vi "data_load_display_trend_fft_mea_coll_v5.vi"() -> ()   [LabVIEW 2020]
uses:
  <vilib>/Utility/file.llb/Read Delimited Spreadsheet (DBL).vi
panel:
  in  "Numeric 2":i32
  out "Waveform Graph 2":dbl[][](graph)
  out "Spectrum plot 2":cluster{i32, dbl, "spectrum out":dbl[]}(graph)
  out "Frequency Interval: delta(f) 2":dbl
  out "xf (frequency) 2":dbl[](array[numeric])
  out "size(s) 2":i32
  out "df (Hz) 2":dbl
  out "ploted signal from each selected frequency 2":dbl[][](graph)
  out "signal from each selected frequency 2":dbl[][](array[numeric])
  out "phase 3":dbl[](array[numeric])
  out "magnitude 3":dbl[](array[numeric])
  out "Numeric 4":i32
  out "Time vs Acceleration graph 2":cluster{"all rows":dbl[], "all rows":dbl[]}(graph)
  out "Acceleration 2":dbl[](array[numeric])
  out "time 2":dbl[](array[numeric])
  out "array w/ subset deleted 2":dbl[][](array[numeric])
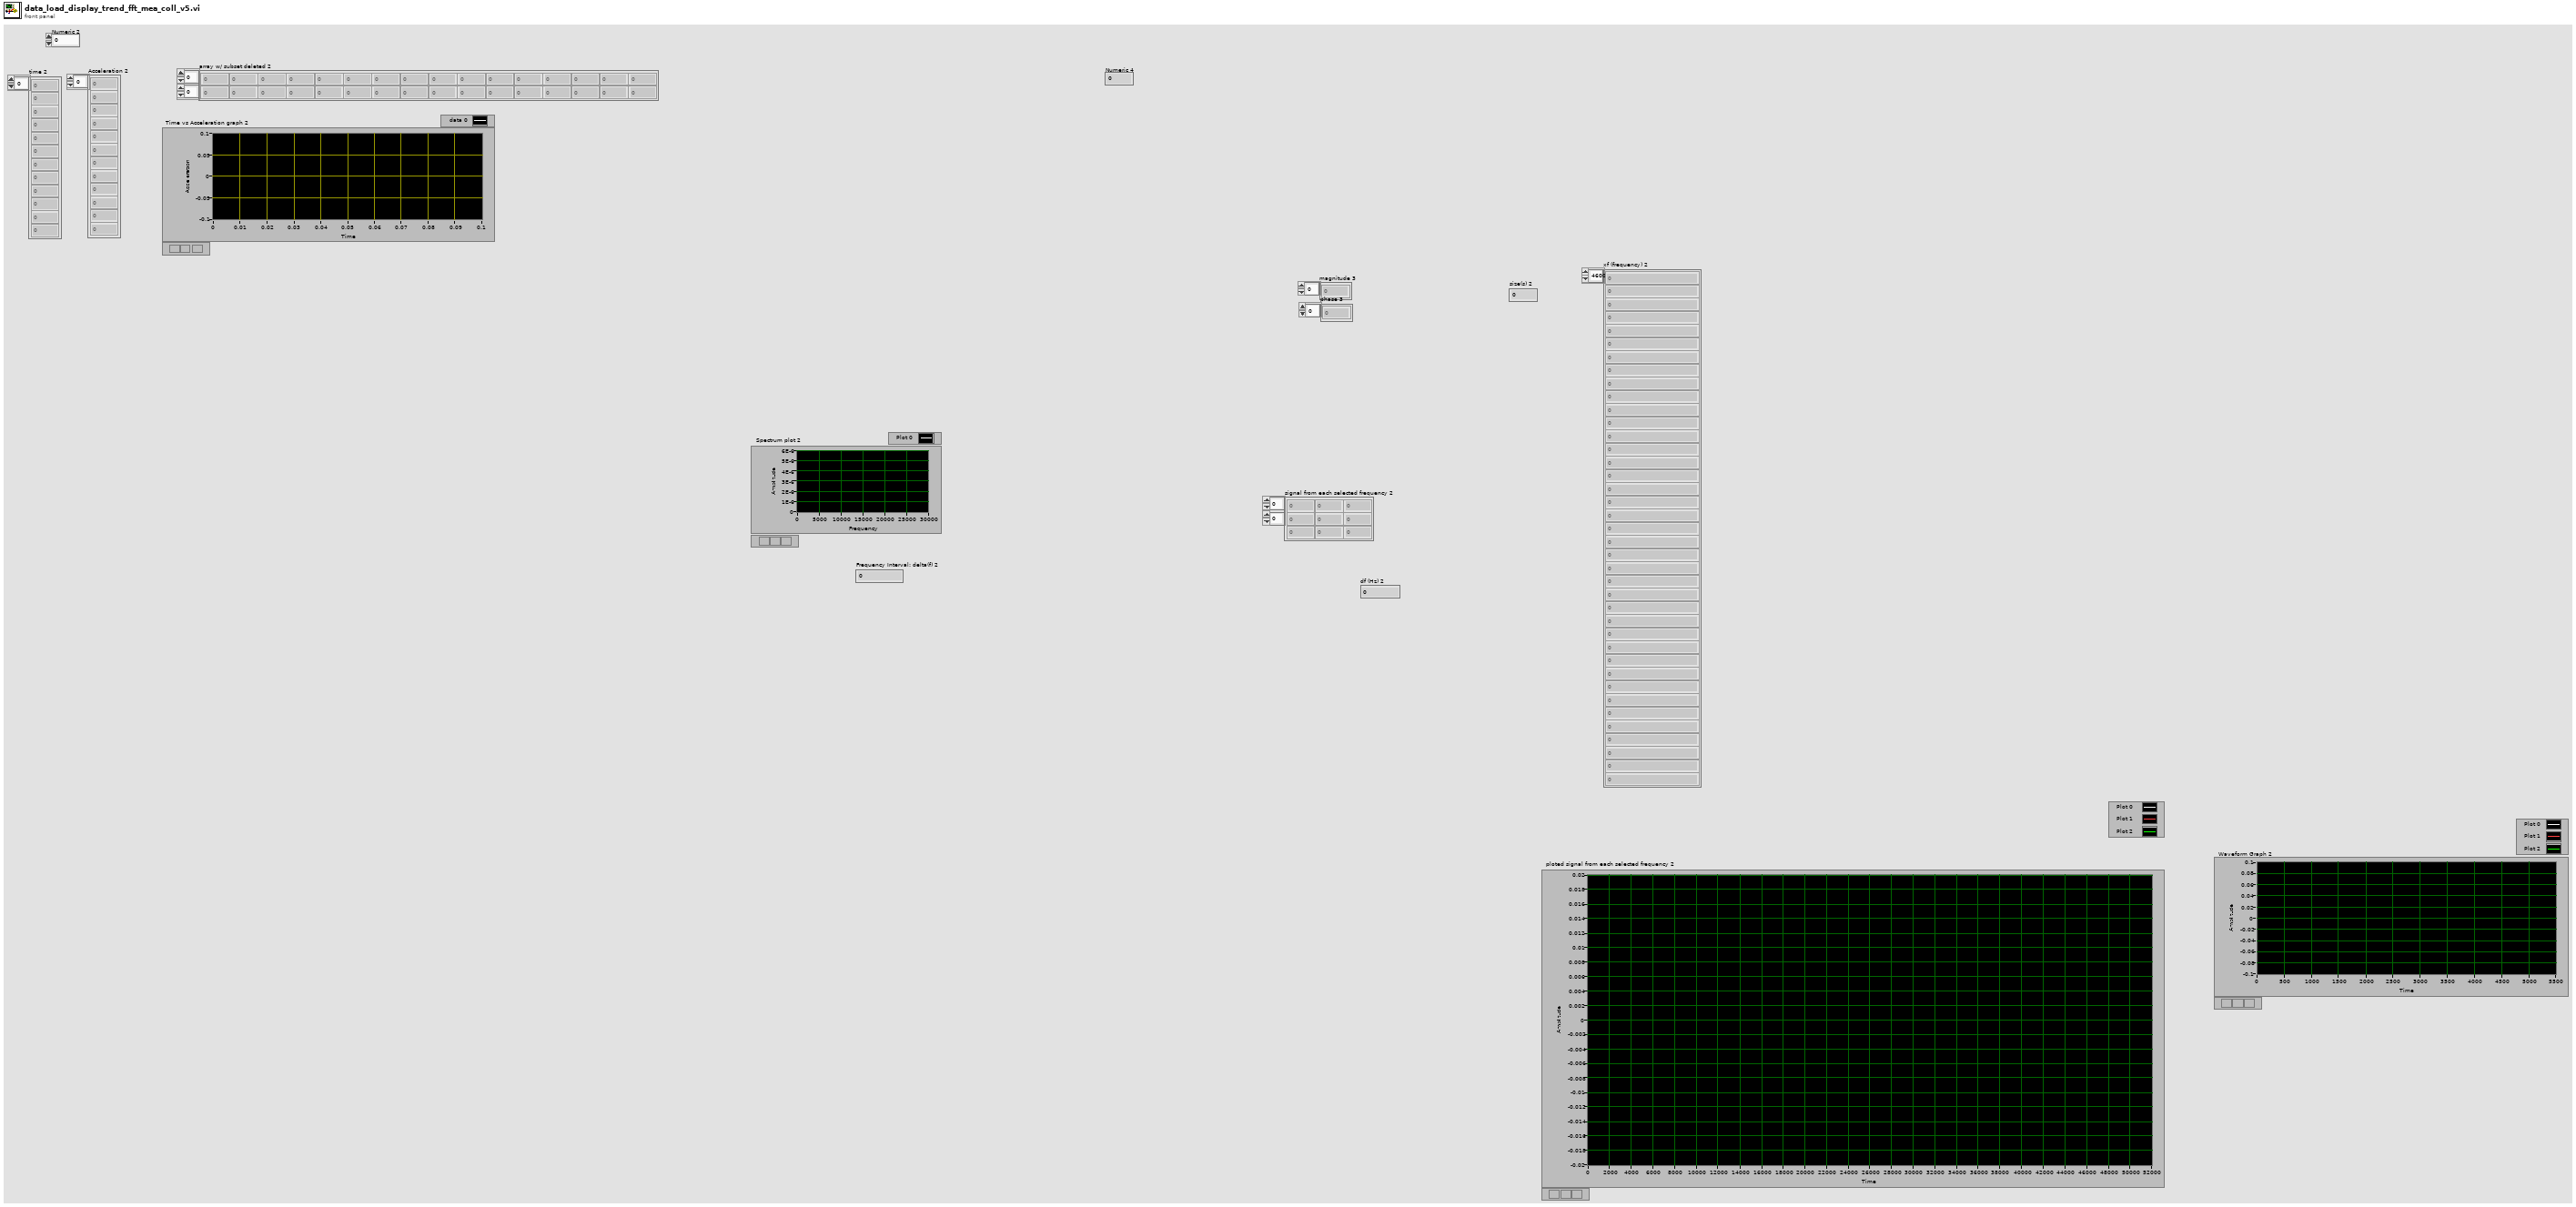
[diagram p1: front panel]
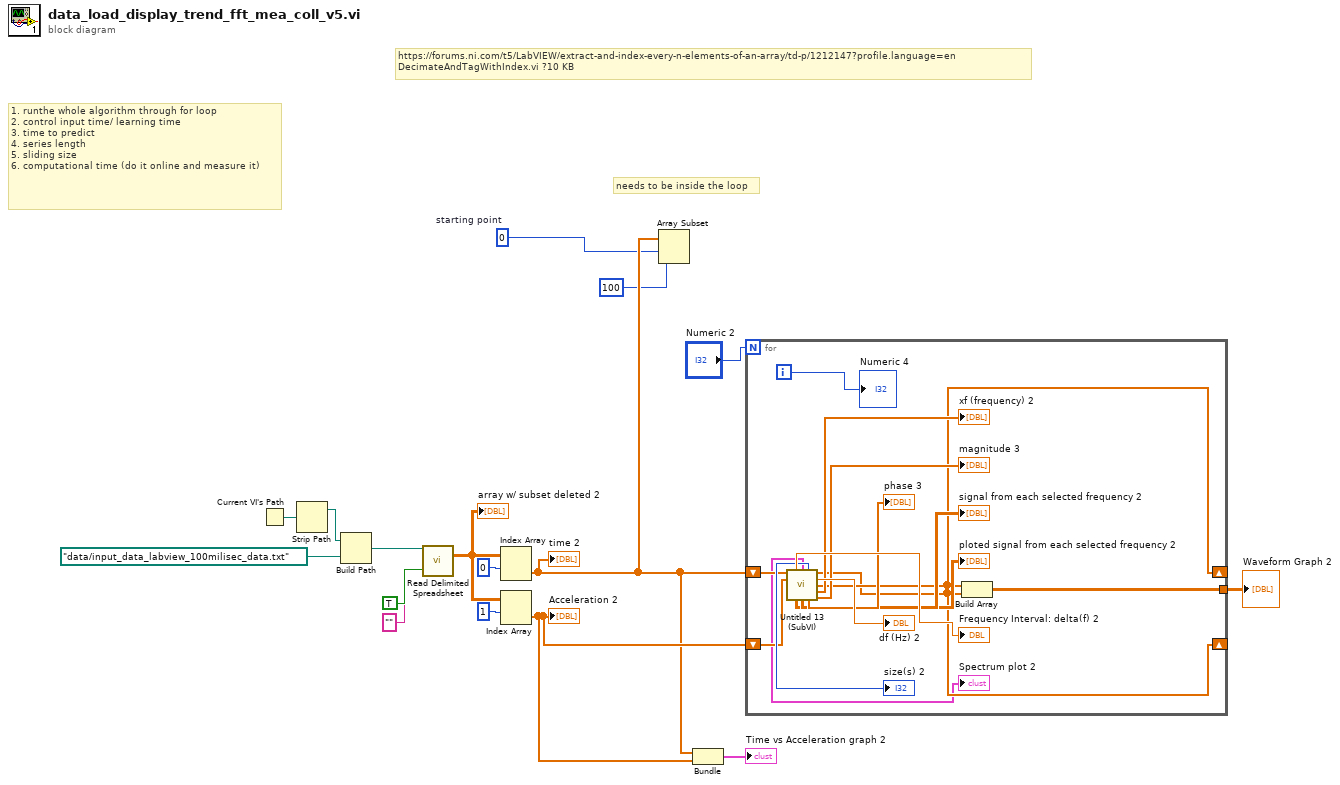
[diagram p0: block diagram]
diagram:
  w2 = 0  # starting point
  # "needs to be inside the loop"
  # "1. runthe whole algorithm through for loop \n2. control input time/ learning time\n3. time to predict\n4. series length\n5. sliding size\n6. computational time (do it online and measure it)"
  # "https://forums.ni.com/t5/LabVIEW/extract-and-index-every-n-elements-of-an-array/td-p/1212147?profile.language=en\nDecimateAndTagWithIndex.vi ?10 KB"
  n1 = Current VI's Path() -> (path=w14:path)
  n2 = Strip Path(path=w14) -> (stripped path=w15:path)  [unwired: 1 out]
  n3 = Build Path(base path=w15, name or relative path=path "data/input_data_labview_100milisec_data.txt") -> (appended path=w16:path)
  n4 = call-poly <vilib>:"Read Delimited Spreadsheet.vi"("file path (dialog if empty)"=w16, "transpose? (F)"=TRUE, "delimiter (\\t)"="" ("delimiter (\\t)")) -> ("all rows"=w13:dbl[][])  [unwired: 7 in, 5 out]
  "array w/ subset deleted 2" <- w13
  n5 = Index Array(array=w13, index (row)=0) -> (element=w3:dbl[])  [unwired: 1 in]
  "time 2" <- w3
  n6 = Index Array(array=w13, index (row)=1) -> (element=w7:dbl[])  [unwired: 1 in]
  "Acceleration 2" <- w7
  n7 = Array Subset(array=w3, index=w2, length=100) -> ()  [unwired: 1 out]
  n8 = Bundle("all rows"=w3, "all rows"=w7) -> (→"Time vs Acceleration graph 2":cluster{"all rows":dbl[], "all rows":dbl[]})  [unwired: 1 in]
  n9 = for {
    N: "Numeric 2" -> [_]
    shift-right: [w20] -> _
    shift-left: w3 -> [w23]
    shift-right: [w19] -> _
    shift-left: w7 -> [w22]
    tunnel: [w21] -> w5
    i -> [w18]
    n10 = call "Untitled 13 (SubVI).vi"(">> time >>"=w23, ">> acceleration >>"=w22) -> ("Frequency Interval: delta(f)"=→"Frequency Interval: delta(f) 2":dbl, "Spectrum plot"=→"Spectrum plot 2":cluster{i32, dbl, "spectrum out":dbl[]}, "size(s)"=→"size(s) 2":i32, "all rows"=w19:dbl[], "df (Hz)"=→"df (Hz) 2":dbl, "Array"=w20:dbl[], "xf (frequency)"=→"xf (frequency) 2":dbl[], "ploted signal from each selected frequency"=→"ploted signal from each selected frequency 2":dbl[][], "signal from each selected frequency"=→"signal from each selected frequency 2":dbl[][], "phase 2"=→"phase 3":dbl[], "magnitude 2"=→"magnitude 3":dbl[])  [unwired: 3 in]
    n11 = Build Array(w20, w19) -> (w21:dbl[][])
    "Numeric 4" <- w18
  }
  "Waveform Graph 2" <- w5
